vi "TimeTag.vi"() -> ()   [LabVIEW 2011]
doc: "This sample project is built upon the standard state machine template and shows how you could create an application that acquires, analyzes, and presents data. It includes functionality for presenting configuration dialogs, preserving settings between executions, loading and saving data, as well as exporting graph images and text files.\n\nIt is most appropriate for data that is acquired instantly as it does not allow for screen updates mid acquisition nor does it allow for continuous streaming to disk."
panel:
  in  "Runs":dbl=100.0
  in  "Pulse TTL 2":bool
  in  "Pulse TTL 1":bool
  in  "Toggle\nTTL 2":bool
  in  "Toggle\nTTL 1":bool
  out "Total Starts":dbl
  in  "Record data":bool
  out "Initial time":dbl
  out "Elapsed time (s)":dbl
  out "FPGA_Run Status":dbl
  out "USB_Open Status":dbl
  out "Channel 4 Total\nCounts":dbl
  out "Channel 3 Total\nCounts":dbl
  out "Channel 2 Total\nCounts":dbl
  out "Channel 1 Total\nCounts":dbl
  in  "File Name":string="C:\\FPGA\\test.txt"
  out "?":dbl
  out "?":dbl
  out "?":dbl
  out "?":dbl
  out "stats":i64[](array[numeric])
  in  "Stop":bool
  out "Channel 4 CPS":dbl(knob) scale=0.0..100000.0
  out "Channel 3 CPS":dbl(knob) scale=0.0..100000.0
  out "Channel 2 CPS":dbl(knob) scale=0.0..100000.0
  out "Channel 1 CPS":dbl(knob) scale=0.0..100000.0
  # "Starts"
  # "Channel 1"
  # "Channel 2"
  # "Channel 3"
  # "Channel 4"
  # "Coincidence Channels 1 & 2"
  # "Coincidence Channels 1 & 3"
  # "Coincidence Channels 1 & 4"
  # "Coincidence Channels 2 & 3"
  # "Coincidence Channels 2 & 4"
  # "Coincidence Channels 3 & 4"
  # "Coincidence Channels 1 & 2 & 3"
  # "Coincidence Channels 1 & 2 & 4"
  # "Coincidence Channels 1 & 3 & 4"
  # "Coincidence Channels 2 & 3 & 4"
  # "Coincidence Channels 1 & 2 & 3 & 4"
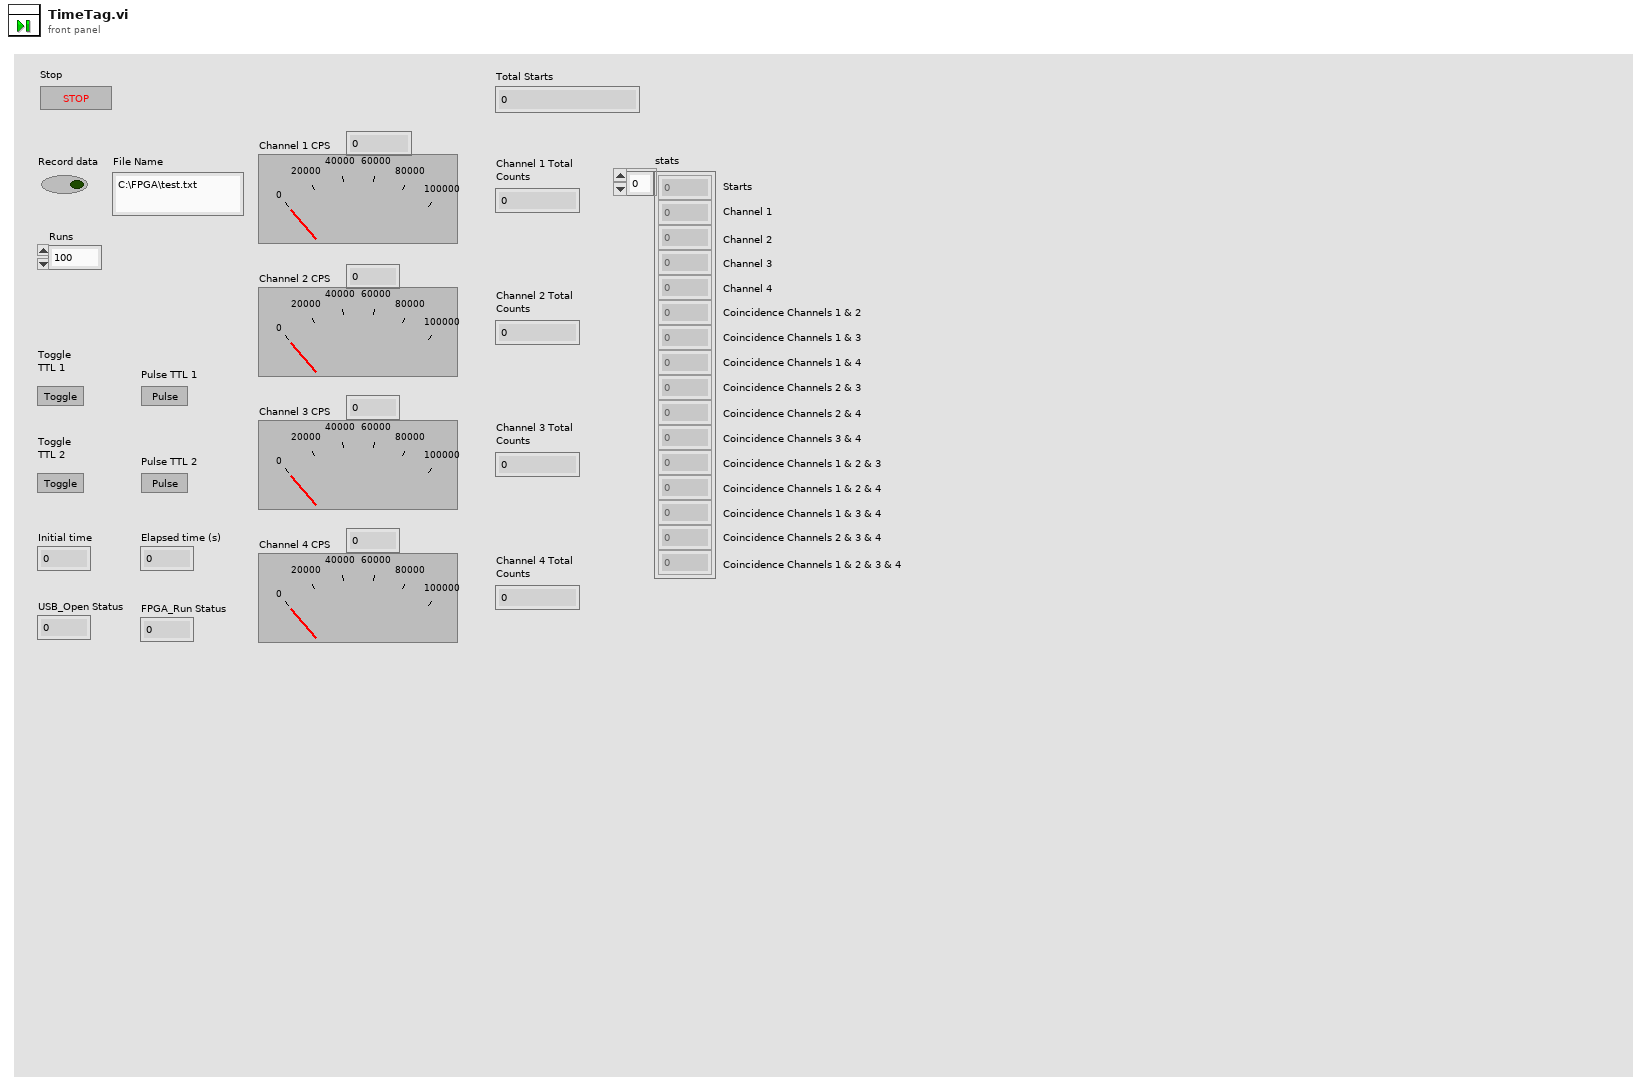
[diagram p1: front panel]
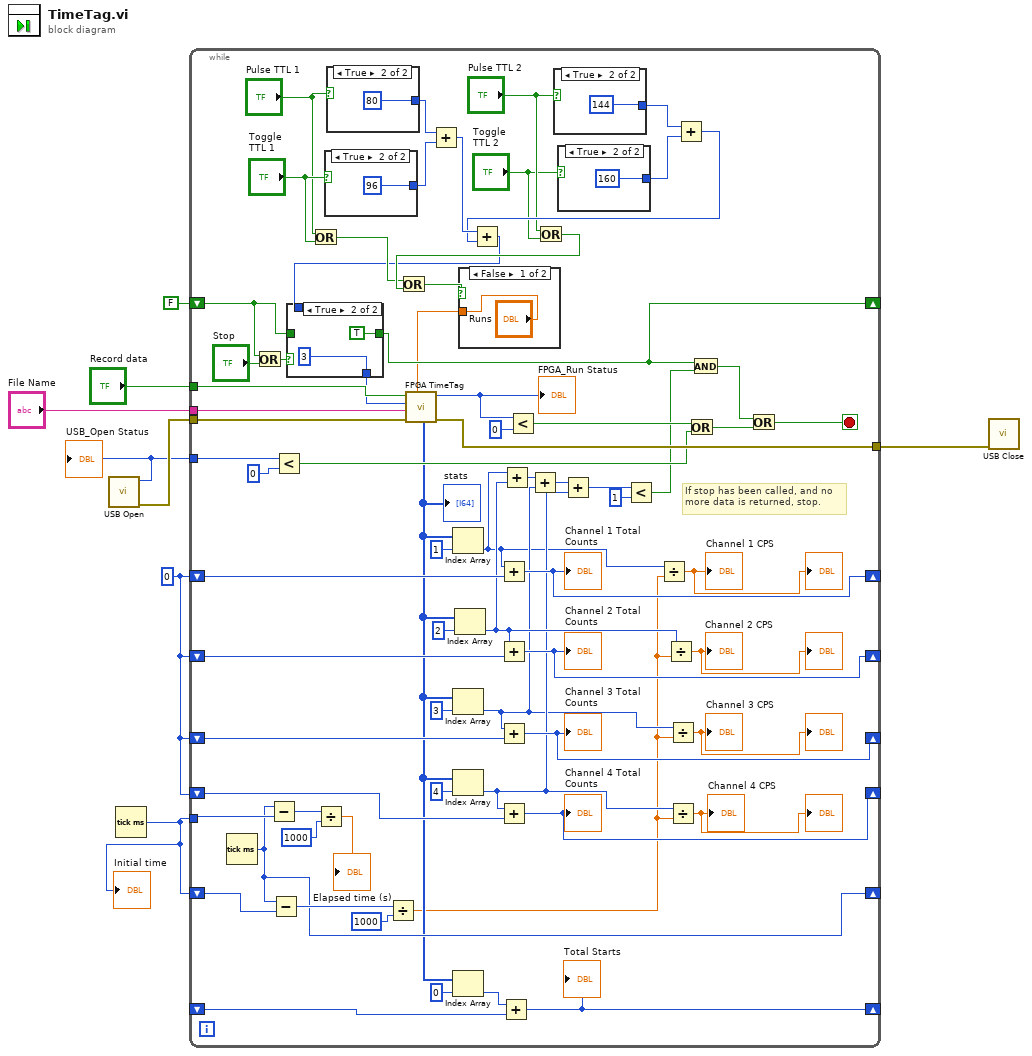
[diagram p0: block diagram]
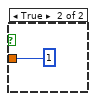
[diagram p2: hidden frame]
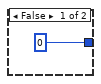
[diagram p3: hidden frame]
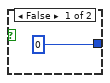
[diagram p4: hidden frame]
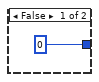
[diagram p5: hidden frame]
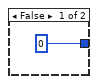
[diagram p6: hidden frame]
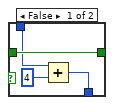
[diagram p7: hidden frame]
diagram:
  w2 = 0
  n1 = call "USB Open.vi"() -> ("error out"=w6:errorcluster, "function return"=w3:i32)  [unwired: 10 in]
  "USB_Open Status" <- w3
  n2 = Tick Count (ms)() -> (millisecond timer value=w4:u32)
  "Initial time" <- w4
  n3 = while {
    tunnel: w4 -> [w80]
    shift-right: [w55] -> _
    shift-left: w2 -> [w50]
    shift-right: [w54] -> _
    shift-left: w2 -> [w49]
    shift-right: [w53] -> _
    shift-left: w2 -> [w48]
    shift-right: [w46] -> _
    shift-left: w2 -> [w47]
    tunnel: w6 -> [w68]
    tunnel: [w69] -> w5
    tunnel: "Record data" -> [w66]
    tunnel: "File Name" -> [w67]
    shift-right: [w51] -> _
    shift-left: w4 -> [w63]
    tunnel: w3 -> [w59]
    shift-right: [w33] -> _
    shift-left: FALSE -> [w30]
    shift-right: [w24] -> _
    shift-left: _ -> [w26]
    stop <- w70 stop-if-true
    # "If stop has been called, and no\nmore data is returned, stop."
    n4 = Tick Count (ms)() -> (millisecond timer value=w51:u32)
    n5 = Or(x=w30, y="Stop") -> (x .or. y?=w32:bool)
    n6 = Subtract(x=w51, y=w80) -> (x-y=w79:u32)
    n7 = Subtract(x=w51, y=w63) -> (x-y=w62:u32)
    n8 = Less?(x=w59, y=0) -> (x < y?=w57:bool)
    n9 = Or(x="Pulse TTL 1", y="Toggle\nTTL 1") -> (x .or. y?=w15:bool)
    n10 = Divide(x=w79, y=1000) -> (x/y=→"Elapsed time (s)":dbl)
    n11 = case shown="True" "Toggle\nTTL 1" {
      tunnel: [0 96] -> w22
      frame False {
      }
      frame True {
      }
    }
    n12 = case shown="True" "Pulse TTL 1" {
      tunnel: [0 80] -> w23
      frame False {
      }
      frame True {
      }
    }
    n13 = Divide(x=w62, y=1000) -> (x/y=w25:dbl)
    n14 = Add(x=w23, y=w22) -> (x+y=w21:i32)
    n15 = Or(x="Pulse TTL 2", y="Toggle\nTTL 2") -> (x .or. y?=w16:bool)
    n16 = Or(x=w15, y=w16) -> (x .or. y?=w17:bool)
    n17 = case shown="False" w17 {
      tunnel: ["Runs" 1] -> w13
      frame False {
      }
      frame True {
      }
    }
    n18 = case shown="True" "Pulse TTL 2" {
      tunnel: [0 144] -> w19
      frame False {
      }
      frame True {
      }
    }
    n19 = case shown="True" "Toggle\nTTL 2" {
      tunnel: [0 160] -> w20
      frame False {
      }
      frame True {
      }
    }
    n20 = Add(x=w19, y=w20) -> (x+y=w18:i32)
    n21 = Add(x=w21, y=w18) -> (x+y=w14:i32)
    n22 = case shown="True" w32 {
      tunnel: [w92 3] -> w52
      tunnel: [w94 TRUE] -> w33
      tunnel: w30 -> [w94 _]
      tunnel: w14 -> [w91 _]
      frame False {
        n23 = Add(x=w91, y=4) -> (x+y=w92:i32)
      }
      frame True {
      }
    }
    n24 = call "FPGA TimeTag.vi"("runs"=w13, "error in (no error)"=w68, "fileName"=w67, "fpgaCommand"=w52, "saveData"=w66) -> ("error out"=w69:errorcluster, "function return"=w65:i32, "stats"=w27:i64[])  [unwired: 4 in]
    "stats" <- w27
    "FPGA_Run Status" <- w65
    n25 = Index Array(array=w27, index=1) -> (element=w36:i64)
    n26 = Index Array(array=w27, index=3) -> (element=w39:i64)
    n27 = Index Array(array=w27, index=4) -> (element=w40:i64)
    n28 = Index Array(array=w27, index=0) -> (element=w28:i64)
    n29 = Index Array(array=w27, index=2) -> (element=w43:i64)
    n30 = Add(x=w36, y=w50) -> (x+y=w55:i64)
    "Channel 1 Total\nCounts" <- w55
    n31 = Add(x=w43, y=w49) -> (x+y=w54:i64)
    "Channel 2 Total\nCounts" <- w54
    n32 = Add(x=w39, y=w48) -> (x+y=w53:i64)
    "Channel 3 Total\nCounts" <- w53
    n33 = Add(x=w40, y=w47) -> (x+y=w46:i64)
    "Channel 4 Total\nCounts" <- w46
    n34 = Add(x=w28, y=w26) -> (x+y=w24:i64)
    "Total Starts" <- w24
    n35 = Add(x=w36, y=w43) -> (x+y=w38:i64)
    n36 = Less?(x=w65, y=0) -> (x < y?=w58:bool)
    n37 = Add(x=w38, y=w39) -> (x+y=w42:i64)
    n38 = Add(x=w42, y=w40) -> (x+y=w41:i64)
    n39 = Less?(x=w41, y=1) -> (x < y?=w35:bool)
    n40 = Divide(x=w36, y=w25) -> (x/y=→"Channel 1 CPS" →"?":dbl)
    n41 = Divide(x=w43, y=w25) -> (x/y=→"Channel 2 CPS" →"?":dbl)
    n42 = Divide(x=w39, y=w25) -> (x/y=→"Channel 3 CPS" →"?":dbl)
    n43 = Divide(x=w40, y=w25) -> (x/y=→"Channel 4 CPS" →"?":dbl)
    n44 = Or(x=w58, y=w57) -> (x .or. y?=w56:bool)
    n45 = And(x=w33, y=w35) -> (x .and. y?=w34:bool)
    n46 = Or(x=w34, y=w56) -> (x .or. y?=w70:bool)
  }
  n47 = call "USB Close.vi"("error in (no error)"=w5) -> ()  [unwired: 9 in, 2 out]
